vi "F Dwf Analog In Status Noise2.vi"(0 "hdwf":i32, 1 "idxData":i32, 5 "idxChannel":i32, 7 "rgdMin":dbl, 9 "rgdMax":dbl, 11 "error in (no error)":errorcluster, 12 "cdData":i32) -> (4 "function return":i32, 8 "rgdMin out":dbl, 10 "rgdMax out":dbl, 15 "error out":errorcluster)   [LabVIEW 2021, in "Olasdwf.lvlib"]
doc: "DWFAPI int FDwfAnalogInStatusNoise2(HDWF hdwf, int idxChannel, double *rgdMin, double *rgdMax, int idxData, int cdData);"
uses:
  Olasdwf.lvlib
  Windows/System32/dwf.dll
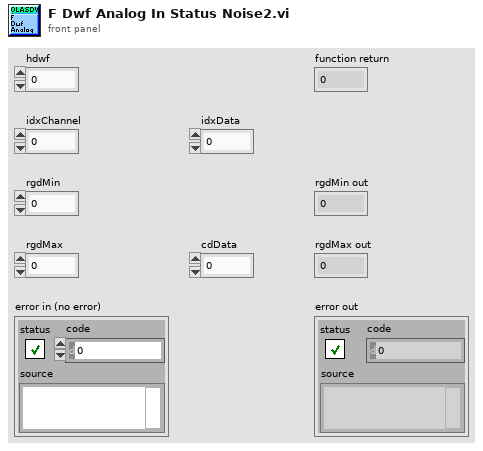
[diagram p1: front panel]
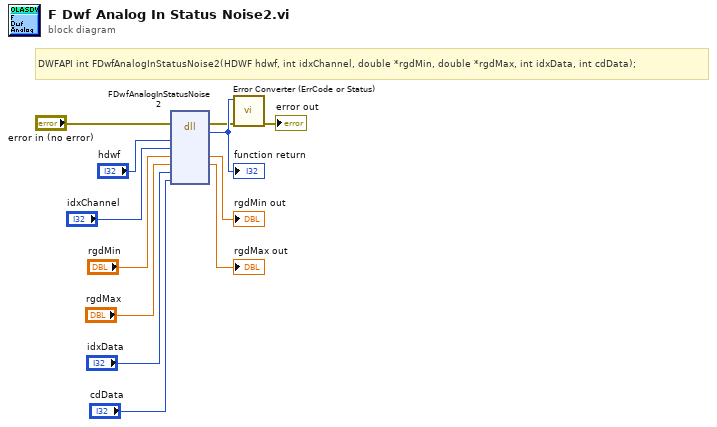
[diagram p0: block diagram]
diagram:
  # "DWFAPI int FDwfAnalogInStatusNoise2(HDWF hdwf, int idxChannel, double *rgdMin, double *rgdMax, int idxData, int cdData);"
  n1 = dll-call lib="/Windows/System32/dwf.*" fn="FDwfAnalogInStatusNoise2"(error in="error in (no error)", "hdwf"="hdwf", "idxChannel"="idxChannel", "rgdMin"="rgdMin", "rgdMax"="rgdMax", "idxData"="idxData", "cdData"="cdData") -> (error out=w2:errorcluster, w12:i32, "rgdMin"=→"rgdMin out":dbl, "rgdMax"=→"rgdMax out":dbl)  [unwired: 6 in, 1 out]
  "function return" <- w12
  n2 = call "Error Converter (ErrCode or Status).vi"("error in (no error)"=w2, "error code"=w12) -> ("error out"=→"error out":errorcluster)  [unwired: 9 in]
